vi "Ctrl.Ring.StyleFont.vi"(8 "error in (no error)":errorcluster, 10 "Font Info":T1, 11 "Ring Ref in":refnum<vi>) -> (0 "error out":errorcluster, 3 "Ring Ref out":refnum<vi>)   [LabVIEW 2020]
uses:
  Font Info -- Cluster.ctl
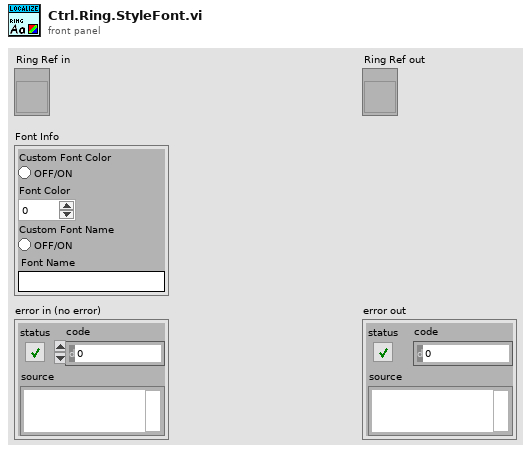
[diagram p1: front panel]
types:
  T1 = typedef "Font Info -- Cluster.ctl" = cluster{"Custom Font Color":bool, "Font Color":u32, "Custom Font Name":bool, "Font Name":string}
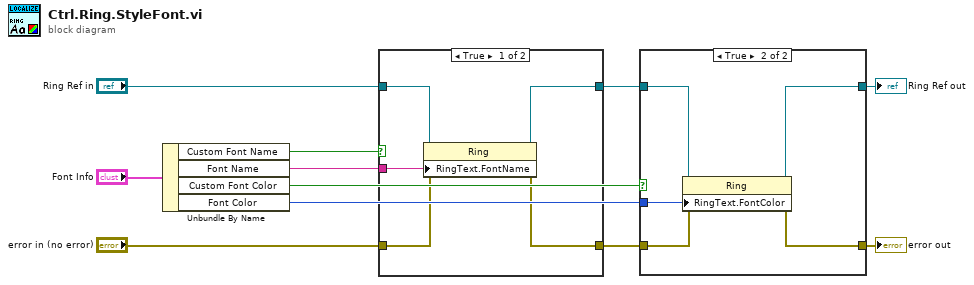
[diagram p0: block diagram]
diagram:
  n1 = Unbundle By Name("Font Info") -> ("Custom Font Name"=w10:bool, "Font Name"=w5:string, "Custom Font Color"=w8:bool, "Font Color"=w4:u32)
  n2 = case shown="True" w10 {
    tunnel: [w13 w17] -> w9
    tunnel: "error in (no error)" -> [w14 w17]
    tunnel: w5 -> [w15 _]
    tunnel: "Ring Ref in" -> [w16 w18]
    tunnel: [w12 w18] -> w2
    frame True {
      n3 = property class="Ring"(reference=w16, error in=w14, "RingText.FontName"=w15) -> (reference out=w12:refnum<vi>, error out=w13:errorcluster)
    }
    frame False {
    }
  }
  n4 = case shown="True" w8 {
    tunnel: w9 -> [w20 w24]
    tunnel: [w20 w23] -> w6
    tunnel: w4 -> [_ w22]
    tunnel: w2 -> [w19 w25]
    tunnel: [w19 w21] -> w1
    frame False {
    }
    frame True {
      n5 = property class="Ring"(reference=w25, error in=w24, "RingText.FontColor"=w22) -> (reference out=w21:refnum<vi>, error out=w23:errorcluster)
    }
  }
  "error out" <- w6
  "Ring Ref out" <- w1
